vi "PPMS_SetCampo.vi"(6 "error in (no error)":errorcluster, 7 "Index":i8) -> (0 "error out":errorcluster, 2 "resulting string 1":string="Set Magnetic Field 1000.000Tesla at 100.000Tesla/min, Linear, Persistent, Sweep&meas", 3 "Cancelled?":bool)   [LabVIEW 2017]
doc: "Use this template to create a dialog box. This template polls the state of the buttons on the front panel and does not use events. Use the Dialog Using Events template (not available in Base package) to create a dialog box with event handling."
panel:
  out "Wait stability":bool=TRUE
  in  "Field Mode":i32(ring) items=["Persistent", "Driven"]
  in  "Approach":i32(ring) items=["Linear", "NoOvershoot", "Oscillate"]
  in  "Rate (Tesla/min)":dbl=0.33
  in  "Campo (Tesla)":dbl=0.5
  in  "Cancel":bool
  in  "OK":bool
  # "Octubre 2019 V1.2  a-sslcdms"
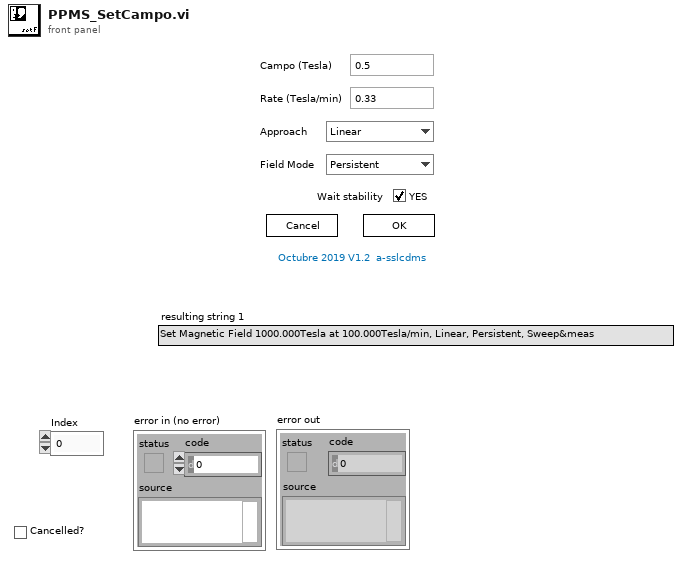
[diagram p1: front panel]
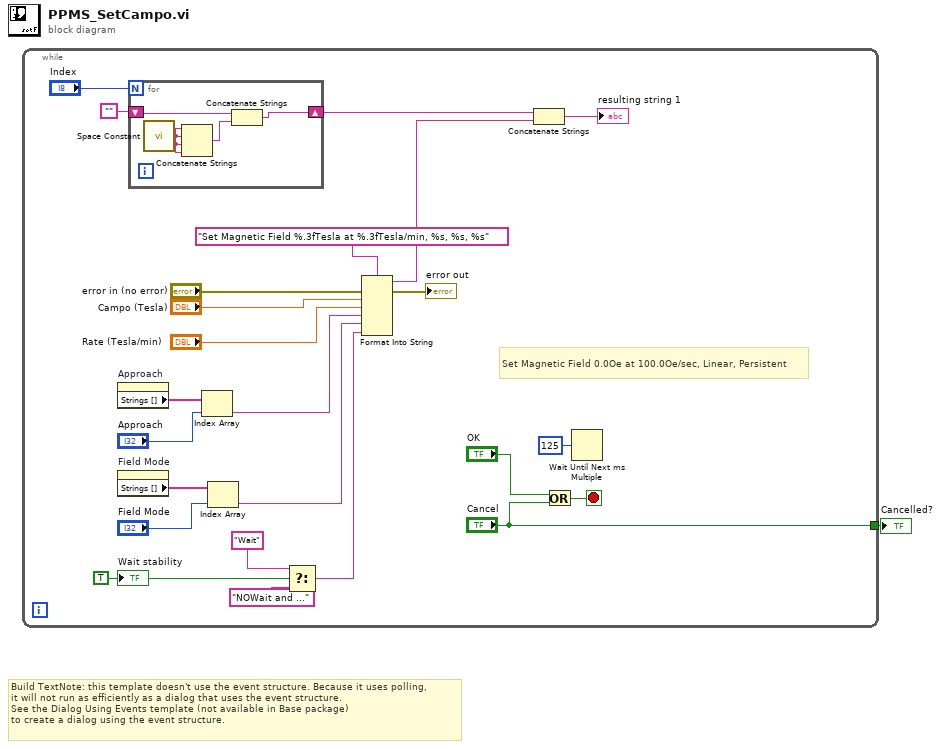
[diagram p0: block diagram]
diagram:
  # "Build TextNote: this template doesn't use the event structure. Because it uses polling, \nit will not run as efficiently as a dialog that uses the event structure.\nSee the Dialog Using Events template (not available in Base package) \nto create a dialog using the event structure."
  n1 = while {
    tunnel: ["Cancel"] -> w1
    stop <- w24 stop-if-true
    w5 = TRUE ("Wait stability")
    # "Set Magnetic Field 0.0Oe at 100.0Oe/sec, Linear, Persistent"
    n2 = property on="Approach" class="Ring (strict)"() -> ("Strings []"=w13:string[])  [unwired: 2 in, 2 out]
    n3 = property on="Field Mode" class="Ring (strict)"() -> ("Strings []"=w9:string[])  [unwired: 2 in, 2 out]
    n4 = for {
      N: "Index" -> [_]
      shift-right: [w28] -> w14
      shift-left: "" -> [w27]
      n5 = call <vilib>:"Space Constant.vi"() -> ("String"=w26:string)
      n6 = Concatenate Strings(w26, w26, w26, w26) -> (w29:string)
      n7 = Concatenate Strings(w27, w29) -> (w28:string)
    }
    n8 = Index Array(array=w13, index="Approach") -> (element=w11:string)
    n9 = Index Array(array=w9, index="Field Mode") -> (element=w7:string)
    n10 = Select(t="Wait", s=w5, f="NOWait and ...") -> (s? t:f=w3:string)
    n11 = Format Into String(format string="Set Magnetic Field %.3fTesla at %.3fTesla/min, %s, %s, %s", error in="error in (no error)", "Campo (Tesla)", "Rate (Tesla/min)", w11, w7, w3) -> (resulting string=w16:string, error out=→"error out":errorcluster)  [unwired: 1 in]
    n12 = Concatenate Strings(w14, w16) -> (→"resulting string 1":string)
    n13 = Or(x="OK", y="Cancel") -> (x .or. y?=w24:bool)
    n14 = Wait Until Next ms Multiple(millisecond multiple=u32 125) -> ()  [unwired: 1 out]
    "Wait stability" <- w5
  }
  "Cancelled?" <- w1
